vi "Microscopy.Acquisition Engine.vi"(0 "Channel Data In":T8=[0, 0, 0, 0], 1 "Engine Commands":T5, 3 "Acquisition Parameters":T9, 9 "Trigger Edges":T6, 11 "Data Valid In":bool) -> (4 "Channel Data Out":T8, 6 "Acquisition Status":T7, 10 "Read Data":bool, 12 "Trigger Output Signals":T4, 13 "Acquisition Debug Status":T3, 14 "Async Frametag Data":T1, 15 "Data Valid Out":bool)   [LabVIEW 2014]
doc: "This VI executes the state machine of the acquisition engine."
uses:
  Acquisition Parameters.ctl
  Adapter Module Specific/Multi-Channel Analog Input Data.ctl
  Acquisition Status.ctl
  Adapter Module Specific/Trigger Signals.ctl
  Adapter Module Specific/Trigger Output Signals.ctl
  Acquisition Engine State.ctl
  Tagging/Async Frametag Data.ctl
panel:
  # "Copyright 2014 Vidrio Technologies\nScanImage 5 software is licensed under the Apache License, Version 2.0 (the \"License\"); you may not use any files contained\nwithin the ScanImage 5 release except in compliance with the License. You may obtain a copy of the License at\n http://www.apache.org/licenses/LICENSE-2.0\nUnless required by applicable law or agreed to in writing, software distributed under the License is distributed on an\n\"AS IS\" BASIS, WITHOUT WARRANTIES OR CONDITIONS OF ANY KIND, either express or implied. See the License for the\n specific language governing permissions and limitations under the License."
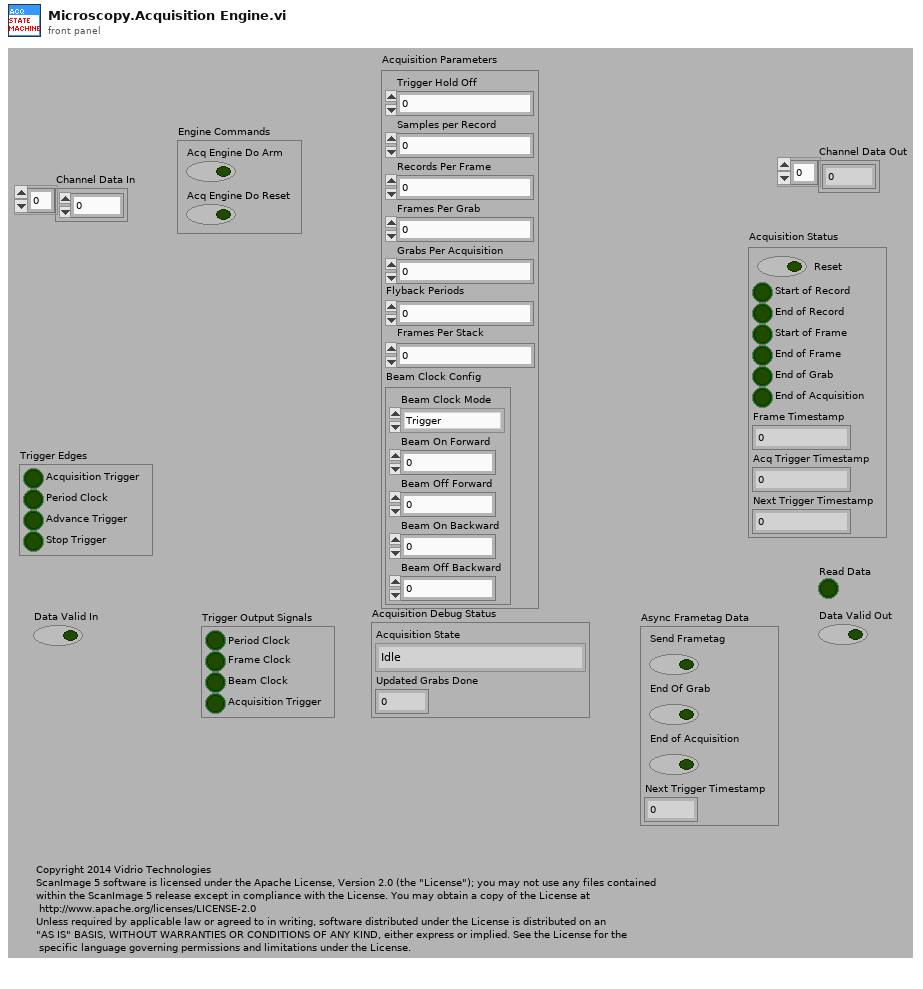
[diagram p1: front panel]
types:
  T1 = typedef "Async Frametag Data.ctl" = cluster{"Send Frametag":bool, "End Of Grab":bool, "End of Acquisition":bool, "Next Trigger Timestamp":u64}
  T2 = typedef "Acquisition Engine State.ctl" = enum8{"Idle", "Wait for Trigger", "Acquisition Hold Off Time", "Read Data", "Check Frame Done", "Check Grab Done", "Check Acquisition Done", "Wait Flyback Periods", "Flush Data"}
  T3 = cluster{"Acquisition State":T2, "Updated Grabs Done":u16}
  T4 = typedef "Trigger Output Signals.ctl" = cluster{"Period Clock":bool, "Frame Clock":bool, "Beam Clock":bool, "Acquisition Trigger":bool}
  T5 = cluster{"Acq Engine Do Arm":bool, "Acq Engine Do Reset":bool}
  T6 = typedef "Trigger Signals.ctl" = cluster{"Acquisition Trigger":bool, "Period Clock":bool, "Advance Trigger":bool, "Stop Trigger":bool}
  T7 = typedef "Acquisition Status.ctl" = cluster{"Reset":bool, "Start of Record":bool, "End of Record":bool, "Start of Frame":bool, "End of Frame":bool, "End of Grab":bool, "End of Acquisition":bool, "Frame Timestamp":u64, "Acq Trigger Timestamp":u64, "Next Trigger Timestamp":u64}
  T8 = typedef "Multi-Channel Analog Input Data.ctl" = i16[]
  T9 = typedef "Acquisition Parameters.ctl" = cluster{"Trigger Hold Off":u16, "Samples per Record":u16, "Records Per Frame":u16, "Frames Per Grab":u32, "Grabs Per Acquisition":u16, "Flyback Periods":u8, "Frames Per Stack":u16, "Beam Clock Config":cluster{"Beam Clock Mode":enum8{"Trigger", "Toggle"}, "Beam On Forward":i16, "Beam Off Forward":i16, "Beam On Backward":i16, "Beam Off Backward":i16}}
  T10 = cluster{"Beam Clock Mode":enum8{"Trigger", "Toggle"}, "Beam On Forward":i16, "Beam Off Forward":i16, "Beam On Backward":i16, "Beam Off Backward":i16}
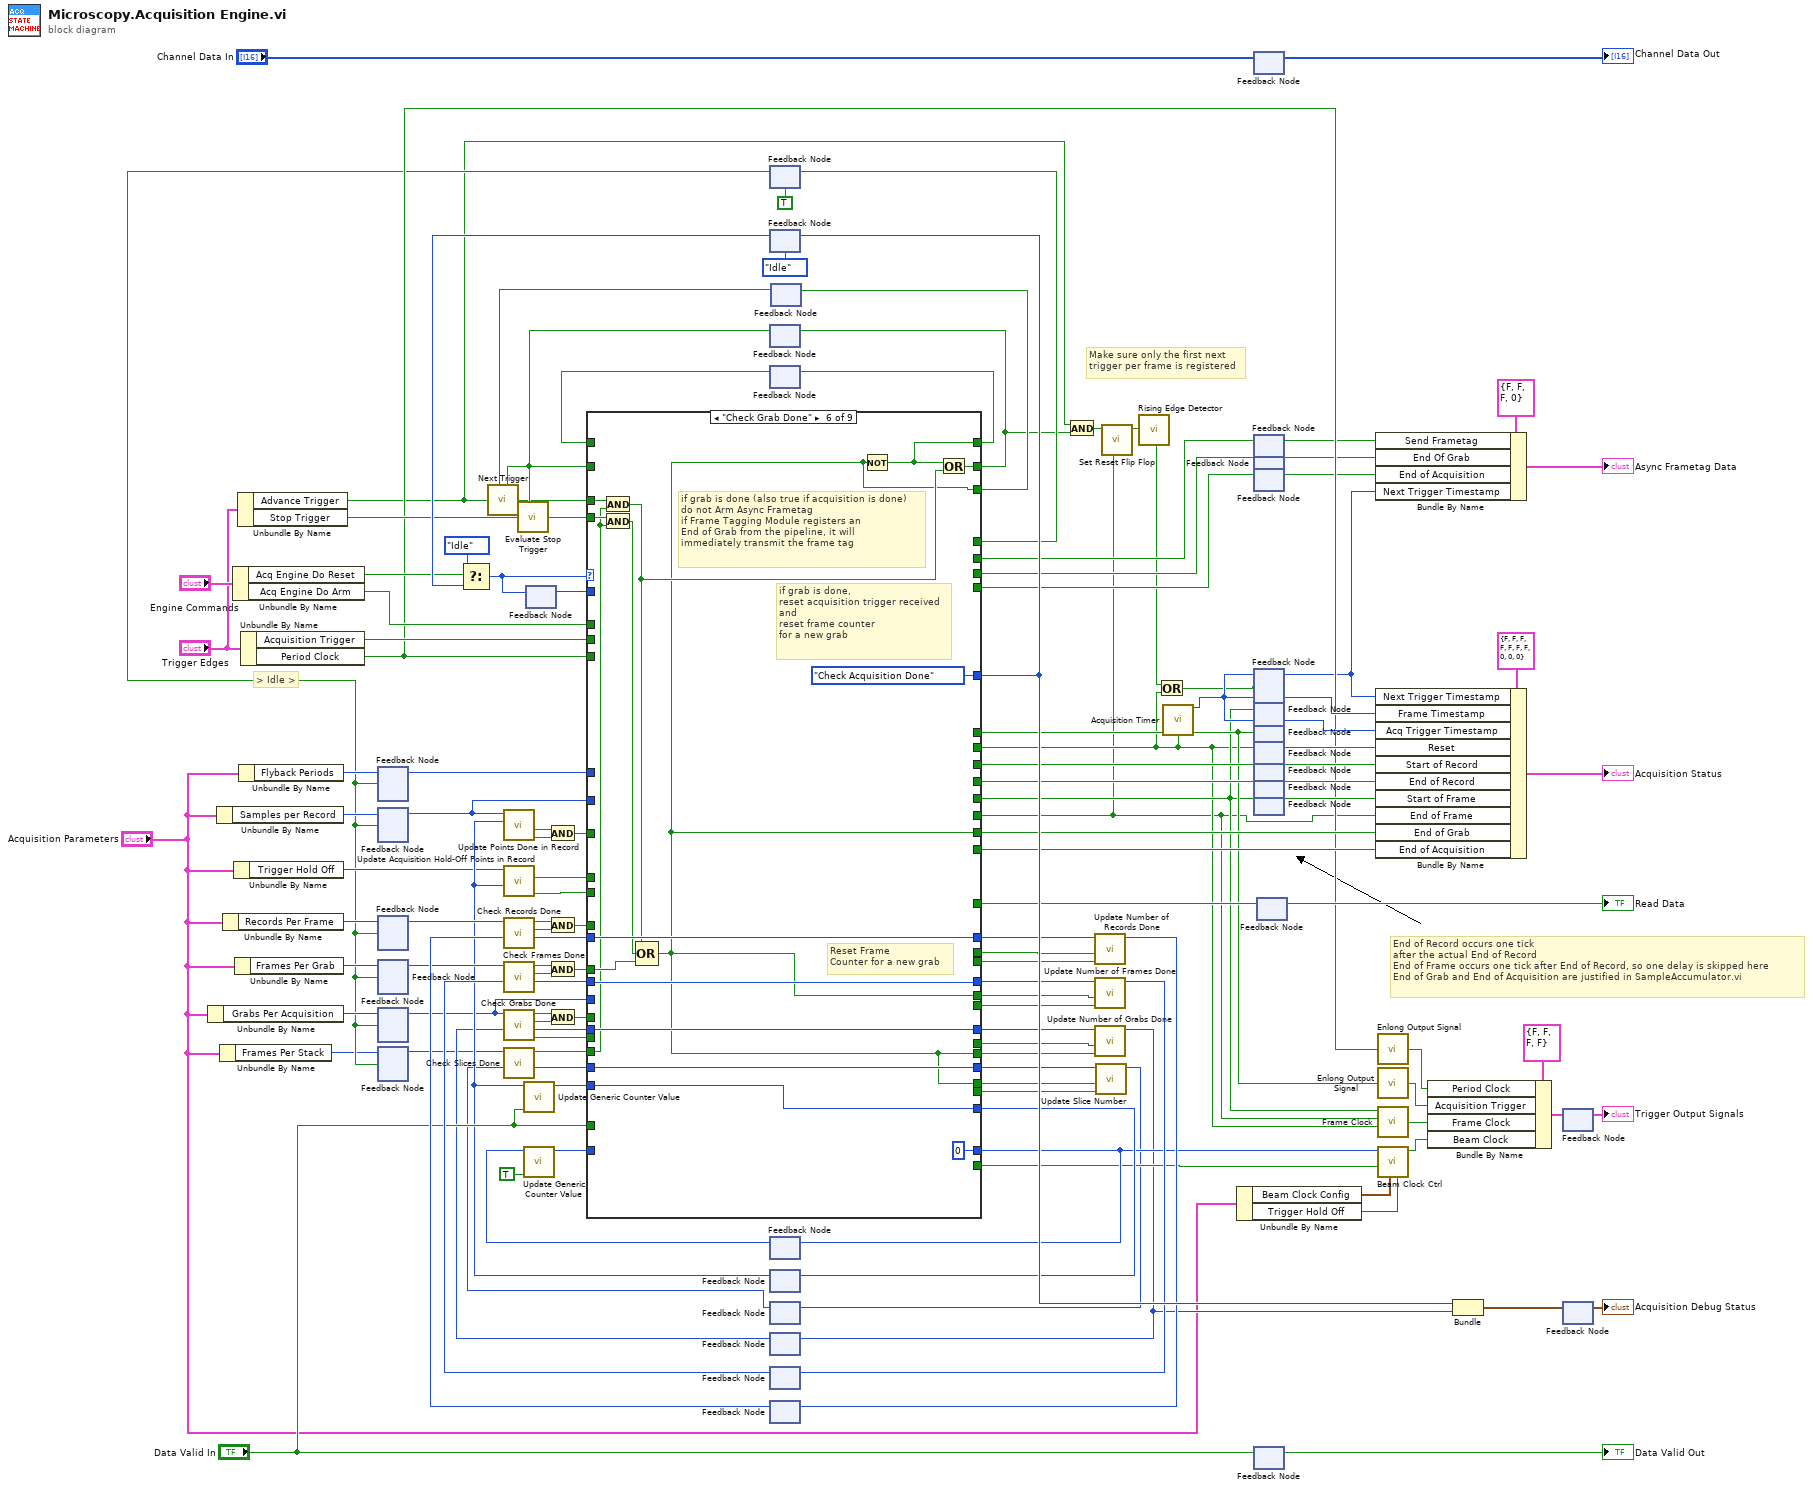
[diagram p0: block diagram]
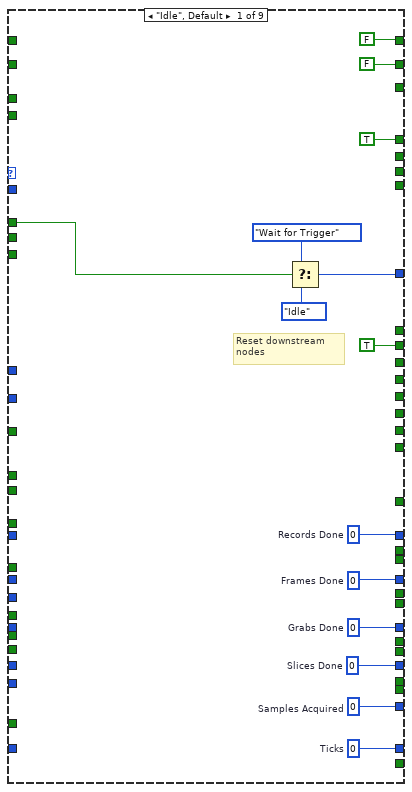
[diagram p2: hidden frame]
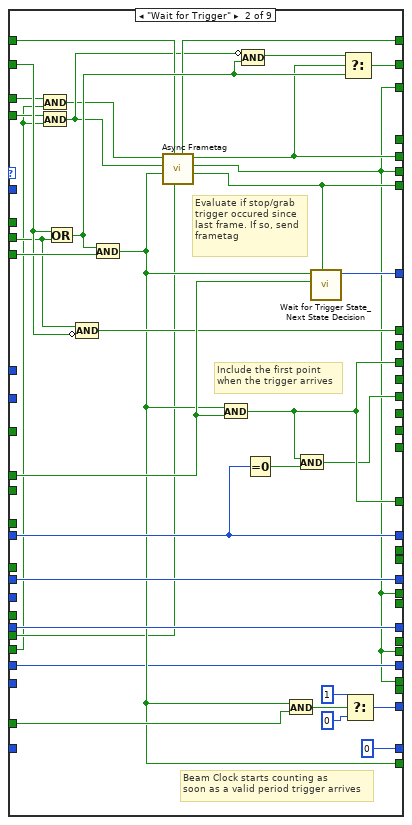
[diagram p3: hidden frame]
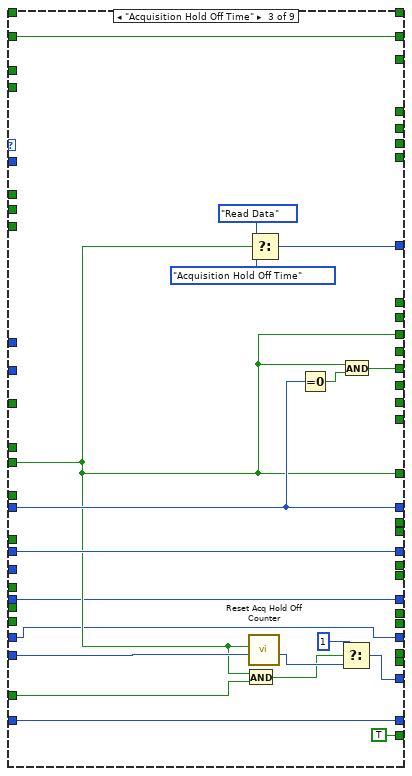
[diagram p4: hidden frame]
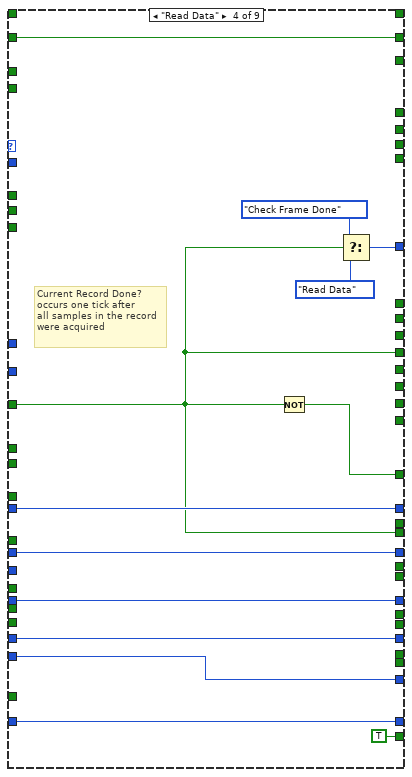
[diagram p5: hidden frame]
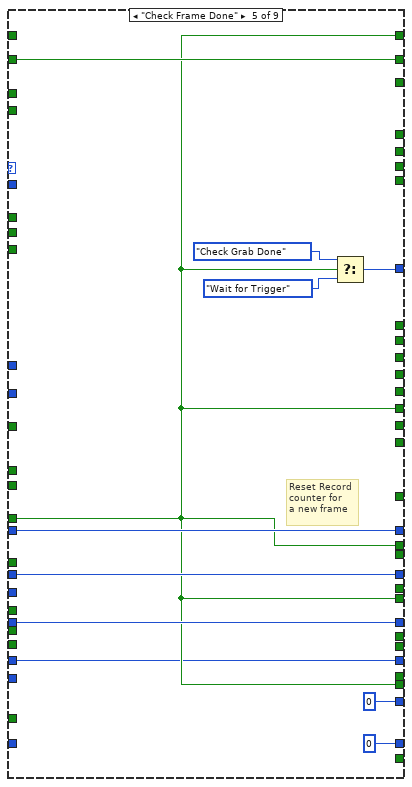
[diagram p6: hidden frame]
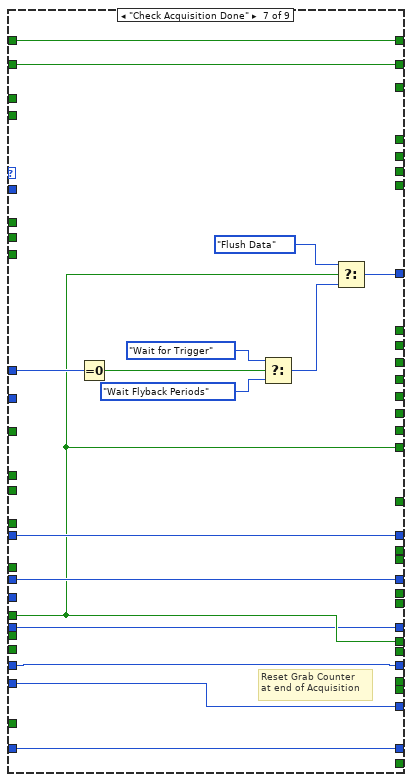
[diagram p7: hidden frame]
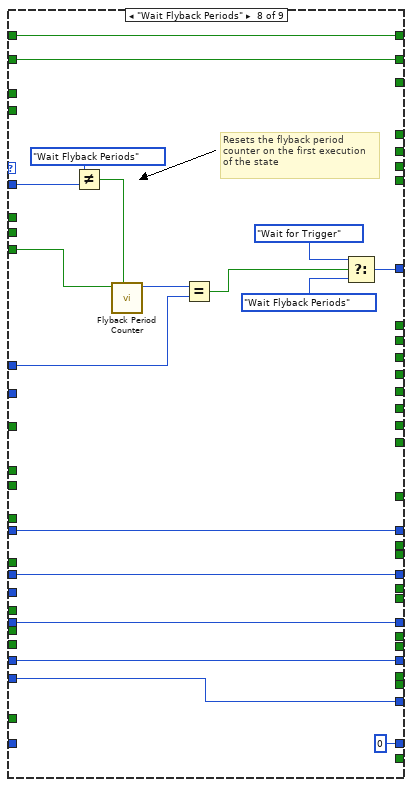
[diagram p8: hidden frame]
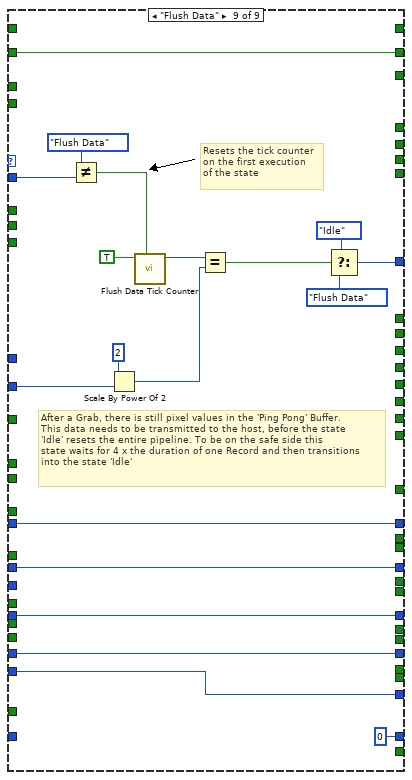
[diagram p9: hidden frame]
diagram:
  # "Make sure only the first next\ntrigger per frame is registered"
  # "> Idle >"
  # "End of Record occurs one tick\nafter the actual End of Record\nEnd of Frame occurs one tick after End of Record, so one delay is skipped here\nEnd of Grab and End of Acquisition are justified in SampleAccumulator.vi"
  n1 = Unbundle By Name("Acquisition Parameters") -> ("Grabs Per Acquisition"=w52:u16)
  n2 = Unbundle By Name("Acquisition Parameters") -> ("Samples per Record"=w108:u16)
  n3 = Unbundle By Name("Acquisition Parameters") -> ("Frames Per Stack"=w9:u16)
  n4 = Unbundle By Name("Acquisition Parameters") -> ("Records Per Frame"=w107:u16)
  n5 = Unbundle By Name("Engine Commands") -> ("Acq Engine Do Reset"=w99:bool, "Acq Engine Do Arm"=w98:bool)
  n6 = Unbundle By Name("Acquisition Parameters") -> ("Trigger Hold Off"=w63:u16)
  n7 = Unbundle By Name("Acquisition Parameters") -> ("Frames Per Grab"=w86:u32)
  n8 = Unbundle By Name("Trigger Edges") -> ("Advance Trigger"=w6:bool, "Stop Trigger"=w54:bool)
  n9 = Unbundle By Name("Acquisition Parameters") -> ("Flyback Periods"=w84:u8)
  n10 = Unbundle By Name("Trigger Edges") -> ("Acquisition Trigger"=w96:bool, "Period Clock"=w47:bool)
  n11 = feedback #1() -> (w83:u8)  [unwired: 1 in]
  n12 = feedback #2() -> (w82:u16)  [unwired: 1 in]
  n13 = feedback #3() -> (w106:u16)  [unwired: 1 in]
  n14 = feedback #4() -> (w85:u32)  [unwired: 1 in]
  n15 = feedback #5() -> (w35:u16)  [unwired: 1 in]
  n16 = feedback #6() -> (w11:u16)  [unwired: 1 in]
  n17 = feedback #7() -> (w78:T2)  [unwired: 1 in]
  n18 = feedback #8(TRUE) -> (w19:bool)
  n19 = feedback-in #1(w84, w19) -> ()
  n20 = feedback-in #2(w108, w19) -> ()
  n21 = feedback-in #3(w107, w19) -> ()
  n22 = feedback-in #4(w86, w19) -> ()
  n23 = feedback-in #5(w52, w19) -> ()
  n24 = feedback-in #6(w9, w19) -> ()
  n25 = feedback #9(Acquisition_Engine_State."Idle" ("f")) -> (w123:T2)
  n26 = Select(t=Acquisition_Engine_State."Idle" ("f"), s=w99, f=w123) -> (s? t:f=w79:T2)
  n27 = feedback-in #7(w79) -> ()
  n28 = feedback #10() -> (w42:bool)  [unwired: 1 in]
  n29 = call "Evaluate Stop Trigger.vi"("Enable"=w42, "Stop Trigger"=w54) -> ("Stop current grab"=w53:bool)  [unwired: 7 in]
  n30 = feedback #11() -> (w36:bool)  [unwired: 1 in]
  n31 = feedback #12() -> (w71:u16)  [unwired: 1 in]
  n32 = call "Update Generic Counter Value.vi"("Increment?"=TRUE, "Input Counter Val"=w71) -> ("Updated Counter Val"=w72:u16)  [unwired: 9 in]
  n33 = feedback #13() -> (w68:u16)  [unwired: 1 in]
  n34 = call "Update Points Done in Record.vi"("Points Acquired"=w68, "Points to Acquire"=w82) -> ("Points Done ?"=w121:bool, "Points to Acquire > 0?"=w116:bool)  [unwired: 7 in, 1 out]
  n35 = call "Update Acquisition Hold-Off Points in Record.vi"("Trigger Hold Off Ticks Finished"=w68, "Trigger Hold-Off Ticks"=w63) -> ("Trigger Hold Off Ticks Finish"=w130:bool, "Is Trigger Hold Off =0?"=w131:bool)  [unwired: 7 in, 1 out]
  n36 = call "Update Generic Counter Value.vi"("Increment?"="Data Valid In", "Input Counter Val"=w68) -> ("Updated Counter Val"=w101:u16)  [unwired: 9 in]
  n37 = And(x=w116, y=w121) -> (x .and. y?=w120:bool)
  n38 = feedback #14() -> (w13:u16)  [unwired: 1 in]
  n39 = call "Check Slices Done.vi"("Slices Done"=w13, "Total Number of Slices"=w11) -> ("Slices Done"=w14:u16, "Stack Done"=w12:bool)  [unwired: 8 in]
  n40 = feedback #15() -> (w56:u16)  [unwired: 1 in]
  n41 = call "Check Grabs Done.vi"("Grabs Finished"=w56, "Grabs to Acquire"=w35) -> ("Next Grab Last"=w34:bool, "Updated Grabs Finished"=w58:u16, "Is NumGrabs >0?"=w60:bool, "Grabs Done?"=w61:bool)  [unwired: 6 in]
  n42 = And(x=w61, y=w60) -> (x .and. y?=w59:bool)
  n43 = feedback #16() -> (w92:u32)  [unwired: 1 in]
  n44 = call "Check Frames Done.vi"("Frames Finished"=w92, "Frames to Acquire"=w85) -> ("Updated Frames Finished"=w91:u32, "Is NumFrames >0?"=w89:bool, "Frames Done?"=w90:bool)  [unwired: 7 in]
  n45 = And(x=w90, y=w89) -> (x .and. y?=w88:bool)
  n46 = feedback #17() -> (w110:u16)  [unwired: 1 in]
  n47 = call "Check Records Done.vi"("Records Finished"=w110, "Records to Acquire"=w106) -> ("Updated Records Finished"=w127:u16, "Is NumRecords >0?"=w118:bool, "Records Done?"=w117:bool)  [unwired: 7 in]
  n48 = And(x=w117, y=w118) -> (x .and. y?=w119:bool)
  n49 = feedback #18() -> (w43:bool)  [unwired: 1 in]
  n50 = call "Next Trigger.vi"("Advance Trigger Reset"=w43, "Advance Trigger in"=w6, "Enable"=w42) -> ("Advance Trigger received"=w5:bool)  [unwired: 6 in]
  n51 = case shown="\"Check Grab Done\"" w79 {
    tunnel: [w149 w163 w202 w214 w224 Acquisition_Engine_State."Check Acquisition Done" ("f") w250 w273 w291] -> w135
    tunnel: w47 -> [_ w183 _ _ _ _ _ w264 _]
    tunnel: w120 -> [_ _ _ w209 _ _ _ _ _]
    tunnel: w98 -> [w145 _ _ _ _ _ _ _ _]
    tunnel: w130 -> [_ _ w189 _ _ _ _ _ _]
    tunnel: w131 -> [_ w182 _ _ _ _ _ _ _]
    tunnel: [w144 w177 w191 w212 w218 w242 w258 w276 w295] -> w129
    tunnel: [_ _ _ w209 _ _ _ _ _] -> w128
    tunnel: w127 -> [_ w177 w191 w212 w218 w242 w258 w276 w295]
    tunnel: w119 -> [_ _ _ _ w217 _ _ _ _]
    tunnel: w101 -> [_ _ w198 w210 _ w241 w257 w275 w294]
    tunnel: [w146 w170 w197 w210 u16 0 ("Updated Records Done") w241 w257 w275 w294] -> w97
    tunnel: [_ w175 w189 w206 _ _ _ _ _] -> w124
    tunnel: [_ w175 w189 _ _ _ _ _ _] -> w122
    tunnel: [_ _ _ w209 _ _ _ _ _] -> w102
    tunnel: w96 -> [_ w172 _ _ _ _ _ _ _]
    tunnel: [TRUE _ _ _ _ _ _ _ _] -> w22
    tunnel: [FALSE w166 w199 w211 w222 w236 w256 w274 w293] -> w4
    tunnel: w42 -> [_ w173 w199 w211 w222 _ w256 w274 w293]
    tunnel: [TRUE _ _ _ _ _ _ _ _] -> w74
    tunnel: "Data Valid In" -> [_ w180 w194 _ _ _ _ _ _]
    tunnel: [w140 w178 w192 w208 w225 w234 w255 w266 w292] -> w95
    tunnel: [_ _ _ _ w217 _ _ _ _] -> w94
    tunnel: w91 -> [_ w178 w192 w208 w225 w234 w255 w266 w292]
    tunnel: w88 -> [_ _ _ _ _ w237 _ _ _]
    tunnel: [_ w174 w188 _ _ _ _ _ _] -> w23
    tunnel: [_ _ _ _ w217 _ _ _ _] -> w1
    tunnel: w83 -> [_ _ _ _ _ _ w249 w270 _]
    tunnel: w82 -> [_ _ _ _ _ _ _ _ w279]
    tunnel: [_ w171 _ _ _ _ _ _ _] -> w80
    tunnel: w78 -> [_ _ _ _ _ _ _ w263 w283]
    tunnel: w72 -> [_ _ w186 w207 _ _ w247 _ _]
    tunnel: [w139 u16 0 ("Updated Counter Val") w186 w207 u16 0 ("Updated Counter Val") u16 0 ("Updated Counter Val") w247 u16 0 ("Updated Counter Val") u16 0 ("Updated Counter Val")] -> w65
    tunnel: [_ w161 TRUE TRUE _ _ _ _ _] -> w64
    tunnel: w59 -> [_ _ _ _ _ _ w245 _ _]
    tunnel: w58 -> [_ w167 w185 w204 w219 w239 w244 w261 w281]
    tunnel: [w138 w167 w185 w204 w219 w239 w244 w261 w281] -> w57
    tunnel: [_ w150 _ _ _ w227 _ _ _] -> w55
    tunnel: w53 -> [_ w156 _ _ _ w231 _ _ _]
    tunnel: [_ _ _ _ _ w227 _ _ _] -> w51
    tunnel: [_ _ _ _ _ _ w245 _ _] -> w50
    tunnel: w5 -> [_ w154 _ _ _ w232 _ _ _]
    tunnel: [_ w150 _ _ _ w227 _ _ _] -> w8
    tunnel: [FALSE w158 _ _ w217 w235 w246 w260 _] -> w37
    tunnel: w36 -> [_ w162 _ _ _ _ w246 w260 _]
    tunnel: [_ w152 _ _ _ _ _ _ _] -> w33
    tunnel: w35 -> [_ _ _ _ _ _ _ _ _]
    tunnel: w34 -> [_ w160 _ _ _ _ _ _ _]
    tunnel: [_ w159 _ _ _ _ _ _ _] -> w32
    tunnel: [_ w150 _ _ _ _ _ _ _] -> w26
    tunnel: [_ w150 _ _ _ w227 _ _ _] -> w25
    tunnel: [_ _ _ _ w217 _ _ _ _] -> w24
    tunnel: [_ _ _ _ _ _ w245 _ _] -> w21
    tunnel: [w136 w157 w184 w203 w216 w233 w243 w259 w277] -> w18
    tunnel: [_ w150 _ _ _ w227 _ _ _] -> w17
    tunnel: [_ _ _ _ w217 _ _ _ _] -> w16
    tunnel: w14 -> [_ w157 w184 w203 w216 w233 w243 w259 w277]
    tunnel: w12 -> [_ w151 _ _ _ w230 _ _ _]
    frame "Idle", Default {
      w136 = u16 0  # Slices Done
      w138 = u16 0  # Grabs Done
      w139 = u16 0  # Ticks
      w144 = u16 0  # Records Done
      w140 = u32 0  # Frames Done
      w146 = u16 0  # Samples Acquired
      # "Reset downstream\nnodes"
      n52 = Select(t=Acquisition_Engine_State."Wait for Trigger" ("f"), s=w145, f=Acquisition_Engine_State."Idle") -> (s? t:f=w149:T2)
    }
    frame "Wait for Trigger" {
      # "Evaluate if stop/grab\ntrigger occured since\nlast frame. If so, send\nframetag"
      # "Beam Clock starts counting as\nsoon as a valid period trigger arrives"
      # "Include the first point\nwhen the trigger arrives"
      n53 = And(x=w154, y=w151) -> (x .and. y?=w153:bool)
      n54 = And(x=w156, y=w151) -> (x .and. y?=w155:bool)
      n55 = Or(x=w173, y=w172) -> (x .or. y?=w164:bool)
      n56 = Compound Arithmetic op=AND(w172, invert w173) -> (w171:bool)
      n57 = And(x=w164, y=w183) -> (x .and. y?=w161:bool)
      n58 = call "Async Frametag.vi"("Last Grab"=w160, "Arm Async Frametag"=w162, "Period Clock received"=w161, "Stop Trigger received"=w155, "Advance Trigger received"=w153) -> ("End of Acquisition"=w159:bool, "End of Grab"=w150:bool, "Send Async Frametag"=w152:bool, "Arm Async Frametag Out"=w158:bool)  [unwired: 3 in]
      n59 = And(x=w161, y=w182) -> (x .and. y?=w175:bool)
      n60 = Compound Arithmetic op=AND(invert w155, w164) -> (w165:bool)
      n61 = Equal To 0?(x=w177) -> (x = 0?=w176:bool)
      n62 = And(x=w161, y=w180) -> (x .and. y?=w179:bool)
      n63 = And(x=w175, y=w176) -> (x .and. y?=w174:bool)
      n64 = call "Wait for Trigger State_Next State Decision.vi"("End of Acquisition"=w159, "Acq Hold=0?"=w182, "Reference Trigger"=w161) -> ("Next State"=w163:T2)  [unwired: 8 in]
      n65 = Select(t=w165, s=w152, f=w164) -> (s? t:f=w166:bool)
      n66 = Select(t=u16 1, s=w179, f=u16 0 ("Updated Records Done")) -> (s? t:f=w170:u16)
    }
    frame "Acquisition Hold Off Time" {
      n67 = And(x=w189, y=w194) -> (x .and. y?=w193:bool)
      n68 = call "Reset Acq Hold Off Counter.vi"("Value"=w198, "Reset"=w189) -> ("Value"=w196:u16)  [unwired: 9 in]
      n69 = Select(t=Acquisition_Engine_State."Read Data" ("f"), s=w189, f=Acquisition_Engine_State."Acquisition Hold Off Time") -> (s? t:f=w202:T2)
      n70 = Equal To 0?(x=w191) -> (x = 0?=w190:bool)
      n71 = Select(t=u16 1 ("Updated Counter Val"), s=w193, f=w196) -> (s? t:f=w197:u16)
      n72 = And(x=w189, y=w190) -> (x .and. y?=w188:bool)
    }
    frame "Read Data" {
      # "Current Record Done?\noccurs one tick after\nall samples in the record\nwere acquired"
      n73 = Not(x=w209) -> (.not. x?=w206:bool)
      n74 = Select(t=Acquisition_Engine_State."Check Frame Done", s=w209, f=Acquisition_Engine_State."Read Data") -> (s? t:f=w214:T2)
    }
    frame "Check Frame Done" {
      # "Reset Record\ncounter for\na new frame"
      n75 = Select(t=Acquisition_Engine_State."Check Grab Done", s=w217, f=Acquisition_Engine_State."Wait for Trigger") -> (s? t:f=w224:T2)
    }
    frame "Check Grab Done" {
      # "if grab is done (also true if acquisition is done)\ndo not Arm Async Frametag\nif Frame Tagging Module registers an\nEnd of Grab from the pipeline, it will\nimmediately transmit the frame tag"
      # "Reset Frame\nCounter for a new grab"
      # "if grab is done,\nreset acquisition trigger received\nand\nreset frame counter\nfor a new grab"
      n76 = And(x=w232, y=w230) -> (x .and. y?=w228:bool)
      n77 = And(x=w231, y=w230) -> (x .and. y?=w229:bool)
      n78 = Compound Arithmetic op=OR(w228, w229, w237) -> (w227:bool)
      n79 = Not(x=w227) -> (.not. x?=w235:bool)
      n80 = Or(x=w235, y=w228) -> (x .or. y?=w236:bool)
    }
    frame "Check Acquisition Done" {
      # "Reset Grab Counter\nat end of Acquisition"
      n81 = Equal To 0?(x=w249) -> (x = 0?=w248:bool)
      n82 = Select(t=Acquisition_Engine_State."Wait for Trigger" ("f"), s=w248, f=Acquisition_Engine_State."Wait Flyback Periods") -> (s? t:f=w251:T2)
      n83 = Select(t=Acquisition_Engine_State."Flush Data" ("f"), s=w245, f=w251) -> (s? t:f=w250:T2)
    }
    frame "Wait Flyback Periods" {
      # "Resets the flyback period\ncounter on the first execution\nof the state"
      n84 = Not Equal?(x=Acquisition_Engine_State."Wait Flyback Periods", y=w263) -> (x != y?=w265:bool)
      n85 = call "Flyback Period Counter.vi"("Reset"=w265, "Period Trigger"=w264) -> ("Periods"=w271:u8)  [unwired: 9 in]
      n86 = Equal?(x=w271, y=w270) -> (x = y?=w268:bool)
      n87 = Select(t=Acquisition_Engine_State."Wait for Trigger" ("x"), s=w268, f=Acquisition_Engine_State."Wait Flyback Periods" ("x")) -> (s? t:f=w273:T2)
    }
    frame "Flush Data" {
      # "Resets the tick counter\non the first execution\nof the state"
      # "After a Grab, there is still pixel values in the 'Ping Pong' Buffer.\nThis data needs to be transmitted to the host, before the state\n'Idle' resets the entire pipeline. To be on the safe side this\nstate waits for 4 x the duration of one Record and then transitions\ninto the state 'Idle'"
      n88 = Not Equal?(x=Acquisition_Engine_State."Flush Data", y=w283) -> (x != y?=w287:bool)
      n89 = Scale By Power Of 2(n=i16 2, x=w279) -> (x*2^n=w278:u16)
      n90 = call "Flush Data Tick Counter.vi"("Reset"=w287, "Increment"=TRUE) -> ("Periods"=w285:u16)  [unwired: 9 in]
      n91 = Equal?(x=w285, y=w278) -> (x = y?=w284:bool)
      n92 = Select(t=Acquisition_Engine_State."Idle" ("f"), s=w284, f=Acquisition_Engine_State."Flush Data") -> (s? t:f=w291:T2)
    }
  }
  n93 = feedback-in #8(w74) -> ()
  n94 = feedback-in #9(w135) -> ()
  n95 = feedback-in #10(w4) -> ()
  n96 = feedback-in #11(w37) -> ()
  n97 = feedback-in #12(w65) -> ()
  n98 = feedback-in #13(w97) -> ()
  n99 = feedback-in #18(w8) -> ()
  n100 = And(x=w6, y=w4) -> (x .and. y?=w3:bool)
  n101 = call "Update Number of Records Done.vi"("Increment?"=w128, "Reset"=w24, "Records Done"=w129) -> ("Updated Records Done"=w109:u16)  [unwired: 8 in]
  n102 = feedback-in #17(w109) -> ()
  n103 = call "Update Number of Frames Done.vi"("Increment?"=w94, "Reset"=w25, "Records Done"=w95) -> ("Updated Records Done"=w93:u32)  [unwired: 8 in]
  n104 = feedback-in #16(w93) -> ()
  n105 = call "Update Number of Grabs Done.vi"("Increment?"=w55, "Reset"=w21, "Grabs Done"=w57) -> ("Updated Grabs Done"=w41:u16)  [unwired: 8 in]
  n106 = feedback-in #15(w41) -> ()
  n107 = call "Update Slice Number.vi"("Increment?"=w16, "Reset"=w17, "Number of Slices"=w18) -> ("Updated Slices Done"=w15:u16)  [unwired: 8 in]
  n108 = feedback-in #14(w15) -> ()
  n109 = call "Set Reset Flip Flop.vi"("Reset"=w1, "Set"=w3) -> ("Out"=w2:bool)  [unwired: 9 in]
  n110 = call "Rising Edge Detector.vi"("signal"=w2) -> ("edge detected"=w7:bool)  [unwired: 14 in]
  n111 = Or(x=w7, y=w22) -> (x .or. y?=w75:bool)
  n112 = call "Acquisition Timer.vi"("Start In"=w80, "Reset"=w22) -> ("Timestamp"=w76:u64, "Start Out"=w49:bool)  [unwired: 12 in]
  n113 = Unbundle By Name("Acquisition Parameters") -> ("Beam Clock Config"=w67:T10, "Trigger Hold Off"=w62:u16)
  n114 = feedback #19() -> (→"Channel Data Out":T8)  [unwired: 1 in]
  n115 = feedback-in #19("Channel Data In") -> ()
  n116 = feedback #20() -> (w29:bool)  [unwired: 1 in]
  n117 = feedback-in #20(w33) -> ()
  n118 = feedback #21() -> (w27:bool)  [unwired: 1 in]
  n119 = feedback-in #21(w26) -> ()
  n120 = feedback #22() -> (w31:bool)  [unwired: 1 in]
  n121 = feedback-in #22(w32) -> ()
  n122 = feedback-in #23(w76, w75) -> ()
  n123 = feedback #23() -> (w30:u64)  [unwired: 1 in]
  n124 = feedback-in #24(w76, w23) -> ()
  n125 = feedback #24() -> (w134:u64)  [unwired: 1 in]
  n126 = feedback-in #25(w76, w49) -> ()
  n127 = feedback #25() -> (w81:u64)  [unwired: 1 in]
  n128 = feedback-in #26(w22) -> ()
  n129 = feedback #26() -> (w114:bool)  [unwired: 1 in]
  n130 = feedback-in #27(w122) -> ()
  n131 = feedback #27() -> (w115:bool)  [unwired: 1 in]
  n132 = feedback-in #28(w102) -> ()
  n133 = feedback #28() -> (w103:bool)  [unwired: 1 in]
  n134 = feedback-in #29(w23) -> ()
  n135 = feedback #29() -> (w87:bool)  [unwired: 1 in]
  n136 = feedback #30() -> (→"Data Valid Out":bool)  [unwired: 1 in]
  n137 = feedback-in #30("Data Valid In") -> ()
  n138 = feedback #31() -> (→"Read Data":bool)  [unwired: 1 in]
  n139 = feedback-in #31(w124) -> ()
  n140 = Bundle By Name(cluster=T1 {"Send Frametag"=FALSE, "End Of Grab"=FALSE, "End of Acquisition"=FALSE, "Next Trigger Timestamp"=0}, "Send Frametag"=w29, "End Of Grab"=w27, "End of Acquisition"=w31, "Next Trigger Timestamp"=w30) -> (→"Async Frametag Data":T1)
  n141 = Bundle By Name(cluster=T7 {"Reset"=FALSE, "Start of Record"=FALSE, "End of Record"=FALSE, "Start of Frame"=FALSE, "End of Frame"=FALSE, "End of Grab"=FALSE, "End of Acquisition"=FALSE, "Frame Timestamp"=0, "Acq Trigger Timestamp"=0, "Next Trigger Timestamp"=0} ("Acquisition Status In"), "Next Trigger Timestamp"=w30, "Frame Timestamp"=w134, "Acq Trigger Timestamp"=w81, "Reset"=w114, "Start of Record"=w115, "End of Record"=w103, "Start of Frame"=w87, "End of Frame"=w1, "End of Grab"=w51, "End of Acquisition"=w50) -> (→"Acquisition Status":T7)
  n142 = call "Enlong Output Signal.vi"("Trigger In"=w47) -> ("Trigger Out"=w46:bool)
  n143 = call "Enlong Output Signal.vi"("Trigger In"=w49) -> ("Trigger Out"=w48:bool)
  n144 = call "Frame Clock.vi"("Start of Frame"=w23, "End of Frame"=w1, "Reset"=w22) -> ("Frame Clock Out"=w20:bool)  [unwired: 4 in]
  n145 = call "Beam Clock Ctrl.vi"("Trigger Hold Off"=w62, "Beam Clock Config"=w67, "Arm"=w64, "Record Ticks"=w65) -> ("Beam Clock"=w66:bool)  [unwired: 7 in]
  n146 = Bundle By Name(cluster=T4 {"Period Clock"=FALSE, "Frame Clock"=FALSE, "Beam Clock"=FALSE, "Acquisition Trigger"=FALSE} ("Trigger Output Signals"), "Period Clock"=w46, "Acquisition Trigger"=w48, "Frame Clock"=w20, "Beam Clock"=w66) -> (w45:T4)
  n147 = Bundle("f"=w135, "Updated Grabs Done"=w41) -> (w40:cluster{"f":T2, "Updated Grabs Done":u16})  [unwired: 1 in]
  n148 = feedback #32() -> (→"Trigger Output Signals":T4)  [unwired: 1 in]
  n149 = feedback-in #32(w45) -> ()
  n150 = feedback #33() -> (→"Acquisition Debug Status":cluster{"f":T2, "Updated Grabs Done":u16})  [unwired: 1 in]
  n151 = feedback-in #33(w40) -> ()
